vi "Dashboard Main.vi"() -> ()   [LabVIEW 2017]
uses:
  <vilib>/Utility/miscctls.llb/LVRowAndColumnTypeDef.ctl
  <vilib>/event_ctls.llb/eventvkey.ctl
  <vilib>/Rock Robotics/Network Tables/NT Read Numeric Array.vi
  <vilib>/Rock Robotics/WPI/Dashboard/WPI_DashboardLogging Global.vi
  <vilib>/Rock Robotics/Network Tables/NT Read Boolean.vi
panel:
  in  "Camera Settings Right":T1={"Frame Rate"=30, "Compression"=30, "Size"=1, "DB Camera Config"=FALSE} {"Frame Rate" scale=1.0..30.0; "Compression" scale=100.0..-1.0; "Size" items=["640x480", "320x240", "160x120"]}
  in  "Camera Name Right":string(combo)="No Camera Selection"
  out "Camera Info":cluster{"Mbps LED":bool, "Mbps":dbl, "fps":dbl} {"fps" format="%#.1g"; "Mbps" format="%#.1g"}
  in  "Camera Settings":T1={"Frame Rate"=30, "Compression"=30, "Size"=1, "DB Camera Config"=FALSE} {"Frame Rate" scale=1.0..30.0; "Compression" scale=100.0..-1.0; "Size" items=["640x480", "320x240", "160x120"]}
  in  "TCP":refnum<k5>
  in  "Rec Mode":enum32{"Stop", "Record", "Playback"}(radio)
  out "Robot IP":string
  out "Image Message":string="Timeout in Camera Communications"
  in  "Dashboard Tab":T2(tab)
  in  "Select Auto":string(combo)="Select Autonomous ..."
  out "NT Connection":bool
  out "MotorChart R":cluster{"Numeric":dbl, "Numeric":dbl}(graph)
  out "MotorChart L":cluster{"Numeric":dbl, "Numeric":dbl}(graph)
  out "MotorSliders R":cluster{"MotorSlide1":dbl, "MotorSlide2":dbl} {"MotorSlide2" scale=-1.0..1.0 scale format="%#_2e"; "MotorSlide1" scale=-1.0..1.0 scale format="%#_2e"}
  out "MotorSliders L":cluster{"MotorSlide1":dbl, "MotorSlide2":dbl} {"MotorSlide2" scale=-1.0..1.0 scale format="%#_2e"; "MotorSlide1" scale=-1.0..1.0 scale format="%#_2e"}
  out "Gyro":dbl(knob) scale=0.0..360.0
  out "JS1 Z":dbl(slide) scale=-1.0..1.0 scale format="%#_2e"
  out "JS1 Graph":cluster{"X":dbl, "Y":dbl}[](graph)
  out "JS1 Buttons":T3
  out "JS2 Z":dbl(slide) scale=-1.0..1.0 scale format="%#_2e"
  out "JS2 Graph":cluster{"X":dbl, "Y":dbl}[](graph)
  out "JS2 Buttons":T3
  out "Mode":T4(ring)=enum."Auto Disabled"
  out "Camera Image Right":T5(plugin-control)
  in  "DB/String 9":string
  in  "DB/String 8":string
  in  "DB/String 7":string
  in  "DB/String 6":string
  in  "DB/String 5":string
  in  "DB/String 4":string
  in  "DB/String 3":string
  in  "DB/String 2":string
  in  "DB/String 1":string
  in  "DB/String 0":string
  in  "DB/Slider 0":dbl(slide) scale=0.0..5.0
  in  "DB/Slider 1":dbl(slide) scale=0.0..5.0
  in  "DB/Slider 2":dbl(slide) scale=0.0..5.0
  in  "DB/Slider 3":dbl(slide) scale=0.0..5.0
  out "DB/LED 3":bool
  out "DB/LED 2":bool
  out "DB/LED 1":bool
  out "DB/LED 0":bool
  in  "DB/Button 3":bool
  in  "DB/Button 2":bool
  in  "DB/Button 1":bool
  in  "DB/Button 0":bool caption="New Name"
  out "Arm Error":string
  out "Has Cube":bool
  in  "Desired Elbow":dbl
  out "Error":string
  out "Shoulder":dbl
  out "Forearm":dbl
  in  "Desired Shoulder":dbl format="%#_13g"
  in  "Solenoid 1/Shoulder":bool
  in  "Solenoid 2/Forearm":bool
  in  "Test Slider":dbl(slide) scale=0.0..100.0 scale format="%#_3g"
  in  "On/Off":bool caption="Solenoid"
  in  "Test Name":u16(ring) items=["Select the test to run..."]
  in  "Test Tree":string(tree)
  in  "Motor":cluster{"Value":dbl, "Enable":bool} {"Value" scale=-1.0..1.0 scale format="%#_3g"}
  out "Progress":T6 {"Test Progress" scale=0.0..100.0}
  in  "Rev/Fwd":cluster{"Forward":bool, "Reverse":bool}
  in  "Test Ring":u16(ring) items=["Monochrome", "Color"]
  out "Cmd Status":string
  in  "Execute Command":bool
  in  "Command Params":string[][](table)
  in  "Command Selection":i32(listbox)
  in  "CheckList":i32(listbox)
  out "Tree":string(tree)
  out "Camera Image":T5(plugin-control)
  out "Background":bool
  in  "Camera Name":string(combo)="No Camera Selection"
  # "HW"
  # "HW"
  # "Joysticks"
  # "Drive Motors"
  # "Front"
  # "Right"
  # "Left"
  # "Back"
  # "This tab is a great place for autonomous settings and robot-specific values.\nPlace controls and indicators inside this tab and match name to\nDashboard Variables on robot. You can also delete this comment."
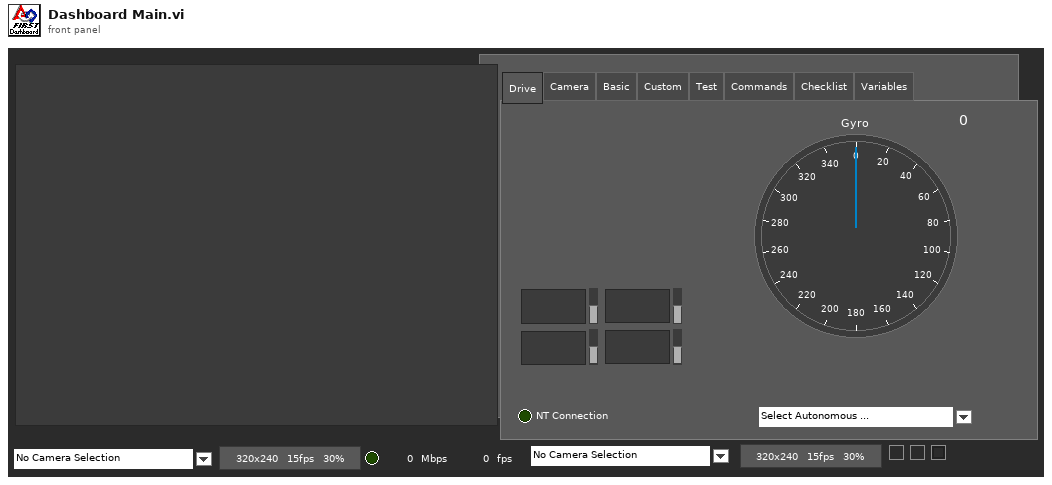
[diagram p1: front panel]
types:
  T1 = cluster{"Frame Rate":i32, "Compression":i32, "Size":u16, "DB Camera Config":bool}
  T2 = enum32{"Drive", "Camera", "Basic", "Custom", "Test", "Commands", "Checklist", "Variables"}
  T3 = cluster{bool, bool, bool, bool, bool, bool, bool, bool, bool, bool, bool, bool}
  T4 = enum8{"Tele-Op Disabled", "Tele-Op Enabled", "Auto Disabled", "Auto Enabled", "Test Disabled", "Test Enabled", "Disconnected", "No Code", "E-Stop"}
  T5 = typedef "IMAQ Image.ctl" = refnum<image>
  T6 = cluster{"Test Progress":u8, "Test Progress Text":string}
  T7 = cluster{"Save Path":path, "Interval (s)":dbl, "Keep":i32}
  T8 = typedef "Image Type" = u32
  T9 = cluster{"IDs":cluster{"RPC field ID":u16, "Unique ID":u16}, "String":string}
  T10 = cluster{"Error Strings":string, "Disable Counts":cluster{u16, u16}, "Rail Faults":cluster{u16, u16, u16}, "Robot IP":string, "DB Mode":u8, "Event Info":cluster{"Name":string, "Type":u8, "Number":u16, "Replay":u8}}
  T11 = cluster{"Storage":cluster{"Disk Free":u64, "RAM Block":u32, "RAM free":u32}, "CPU Utilization":cluster{"CPU % ISR":sgl, "CPU % Time Crit":sgl, "CPU % Timed Str":sgl, "CPU % High":sgl, "CPU % Above":sgl, "CPU % Normal":sgl, "CPU % Low":sgl}, "CAN":cluster{"% Bus Utilization":sgl, "Bus Off Cnt":u32, "TX_FIFO Full Cnt":u32, "Receive Error Cnt":u8, "Transmit Error Cnt":u8}, "HID":cluster{"HID Outputs":u32, "Rumble Low":u16, "Rumble High":u16}[]}
  T12 = cluster{"Status bits":cluster{"Test Mode":bool, "Autonomous":bool, "Enabled":bool, "Code Start":bool, "Brownout":bool, "Reserved 2":bool, "Reserved 3":bool, "E-Stop":bool}, "Code Trace":cluster{"Disabled":bool, "TeleOp":bool, "Auto":bool, "Test":bool}, "Controller Type":enum16{"unknown", "cRIO", "roboRio"}, "Code?":enum16{"unknown", "noCode", "code"}, "Battery V":dbl}
  T13 = cluster{"Control Bits":cluster{"TestMode":bool, "Autonomous":bool, "Enabled":bool, "FMS Present":bool, bool, bool, bool, "E-Stop":bool}, "Team Station ":u8, "Countdown":sgl, "Joystick Values":cluster{"Axes":dbl[], "Buttons":bool[], "POVs":i16[]}[]}
  T14 = cluster{"Axes":dbl[], "Buttons":bool[], "POVs":i16[]}[]
  T15 = cluster{"Axes":dbl[], "Buttons":bool[], "POVs":i16[]}
  T16 = cluster{"Buttons[0]":bool, "Buttons[1]":bool, "Buttons[2]":bool, "Buttons[3]":bool, "Buttons[4]":bool, "Buttons[5]":bool, "Buttons[6]":bool, "Buttons[7]":bool, "Buttons[8]":bool, "Buttons[9]":bool, "Buttons[10]":bool, "Buttons[11]":bool}
  T17 = cluster{"Camera Image":refnum<vi>, "Dashboard Tab":refnum<vi>, "Background":refnum<vi>, "Rec Mode":refnum<vi>, "Test Slider":refnum<vi>, "On/Off ":refnum<vi>, "Test Ring":refnum<vi>, "Rev/Fwd":refnum<vi>, "Test Name":refnum<vi>, "Motor":refnum<vi>, "Progress":refnum<vi>, "CheckList":refnum<vi>, "Tree":refnum<vi>, "Test Tree":refnum<vi>, "Command Params":refnum<vi>, "Command Selection":refnum<vi>, "Execute Command":refnum<vi>, "Cmd Status":refnum<vi>, "Camera Settings":refnum<vi>, "Camera Name":refnum<vi>, "Camera Info":refnum<vi>, "Camera Settings Right":refnum<vi>, "Camera Name Right":refnum<vi>, "Camera Image Right":refnum<vi>}
  T18 = cluster{"Camera Name Right":string, string, "Saved DB Images Info":cluster{"Save Path":path, "Interval (s)":dbl, "Keep":i32}}
  T19 = cluster{"Camera Name":string, string, "Saved DB Images Info":cluster{"Save Path":path, "Interval (s)":dbl, "Keep":i32}}
  T20 = cluster{"Operation":enum16{"Update", "Clear"}, "Color Box":u32}[]
  T21 = typedef "eventvkey.ctl" = enum16{"ASCII", "Enter", "Return", "Shift", "Ctrl", "Alt", "Cmd", "Opt", "Caps", "NumLock", "Clear", "Break", "Up", "Down", "Left", "Right", "Insert", "Delete", "Home", "End", "PageUp", "PageDown", "Escape", "Help", "Pause", "ScrollLock", "F1", "F2", "F3", "F4", "F5", "F6", "F7", "F8", "F9", "F10", "F11", "F12", "F13", "F14", "F15", "F16", "F17", "F18", "F19", "F20", "F21", "F22", "F23", "F24", "Play", "VolumeUp", "VolumeDown", "Mute", "Two Byte Char"}
  T22 = cluster{"Image Size":bool, "Image Type":bool, "Pixel Value":bool, "ROI Information":bool, "Zoom Factor":bool}
  T23 = cluster{"Operation":enum16{"Update", "Clear"}, "Color Box":u32}
  T24 = typedef "LVRowAndColumnTypeDef.ctl" = cluster{"Row":i32, "Column":i32}
  T25 = cluster{"Shift":bool, "Ctrl":bool, "Alt":bool, "Cmd":bool, "Opt":bool}
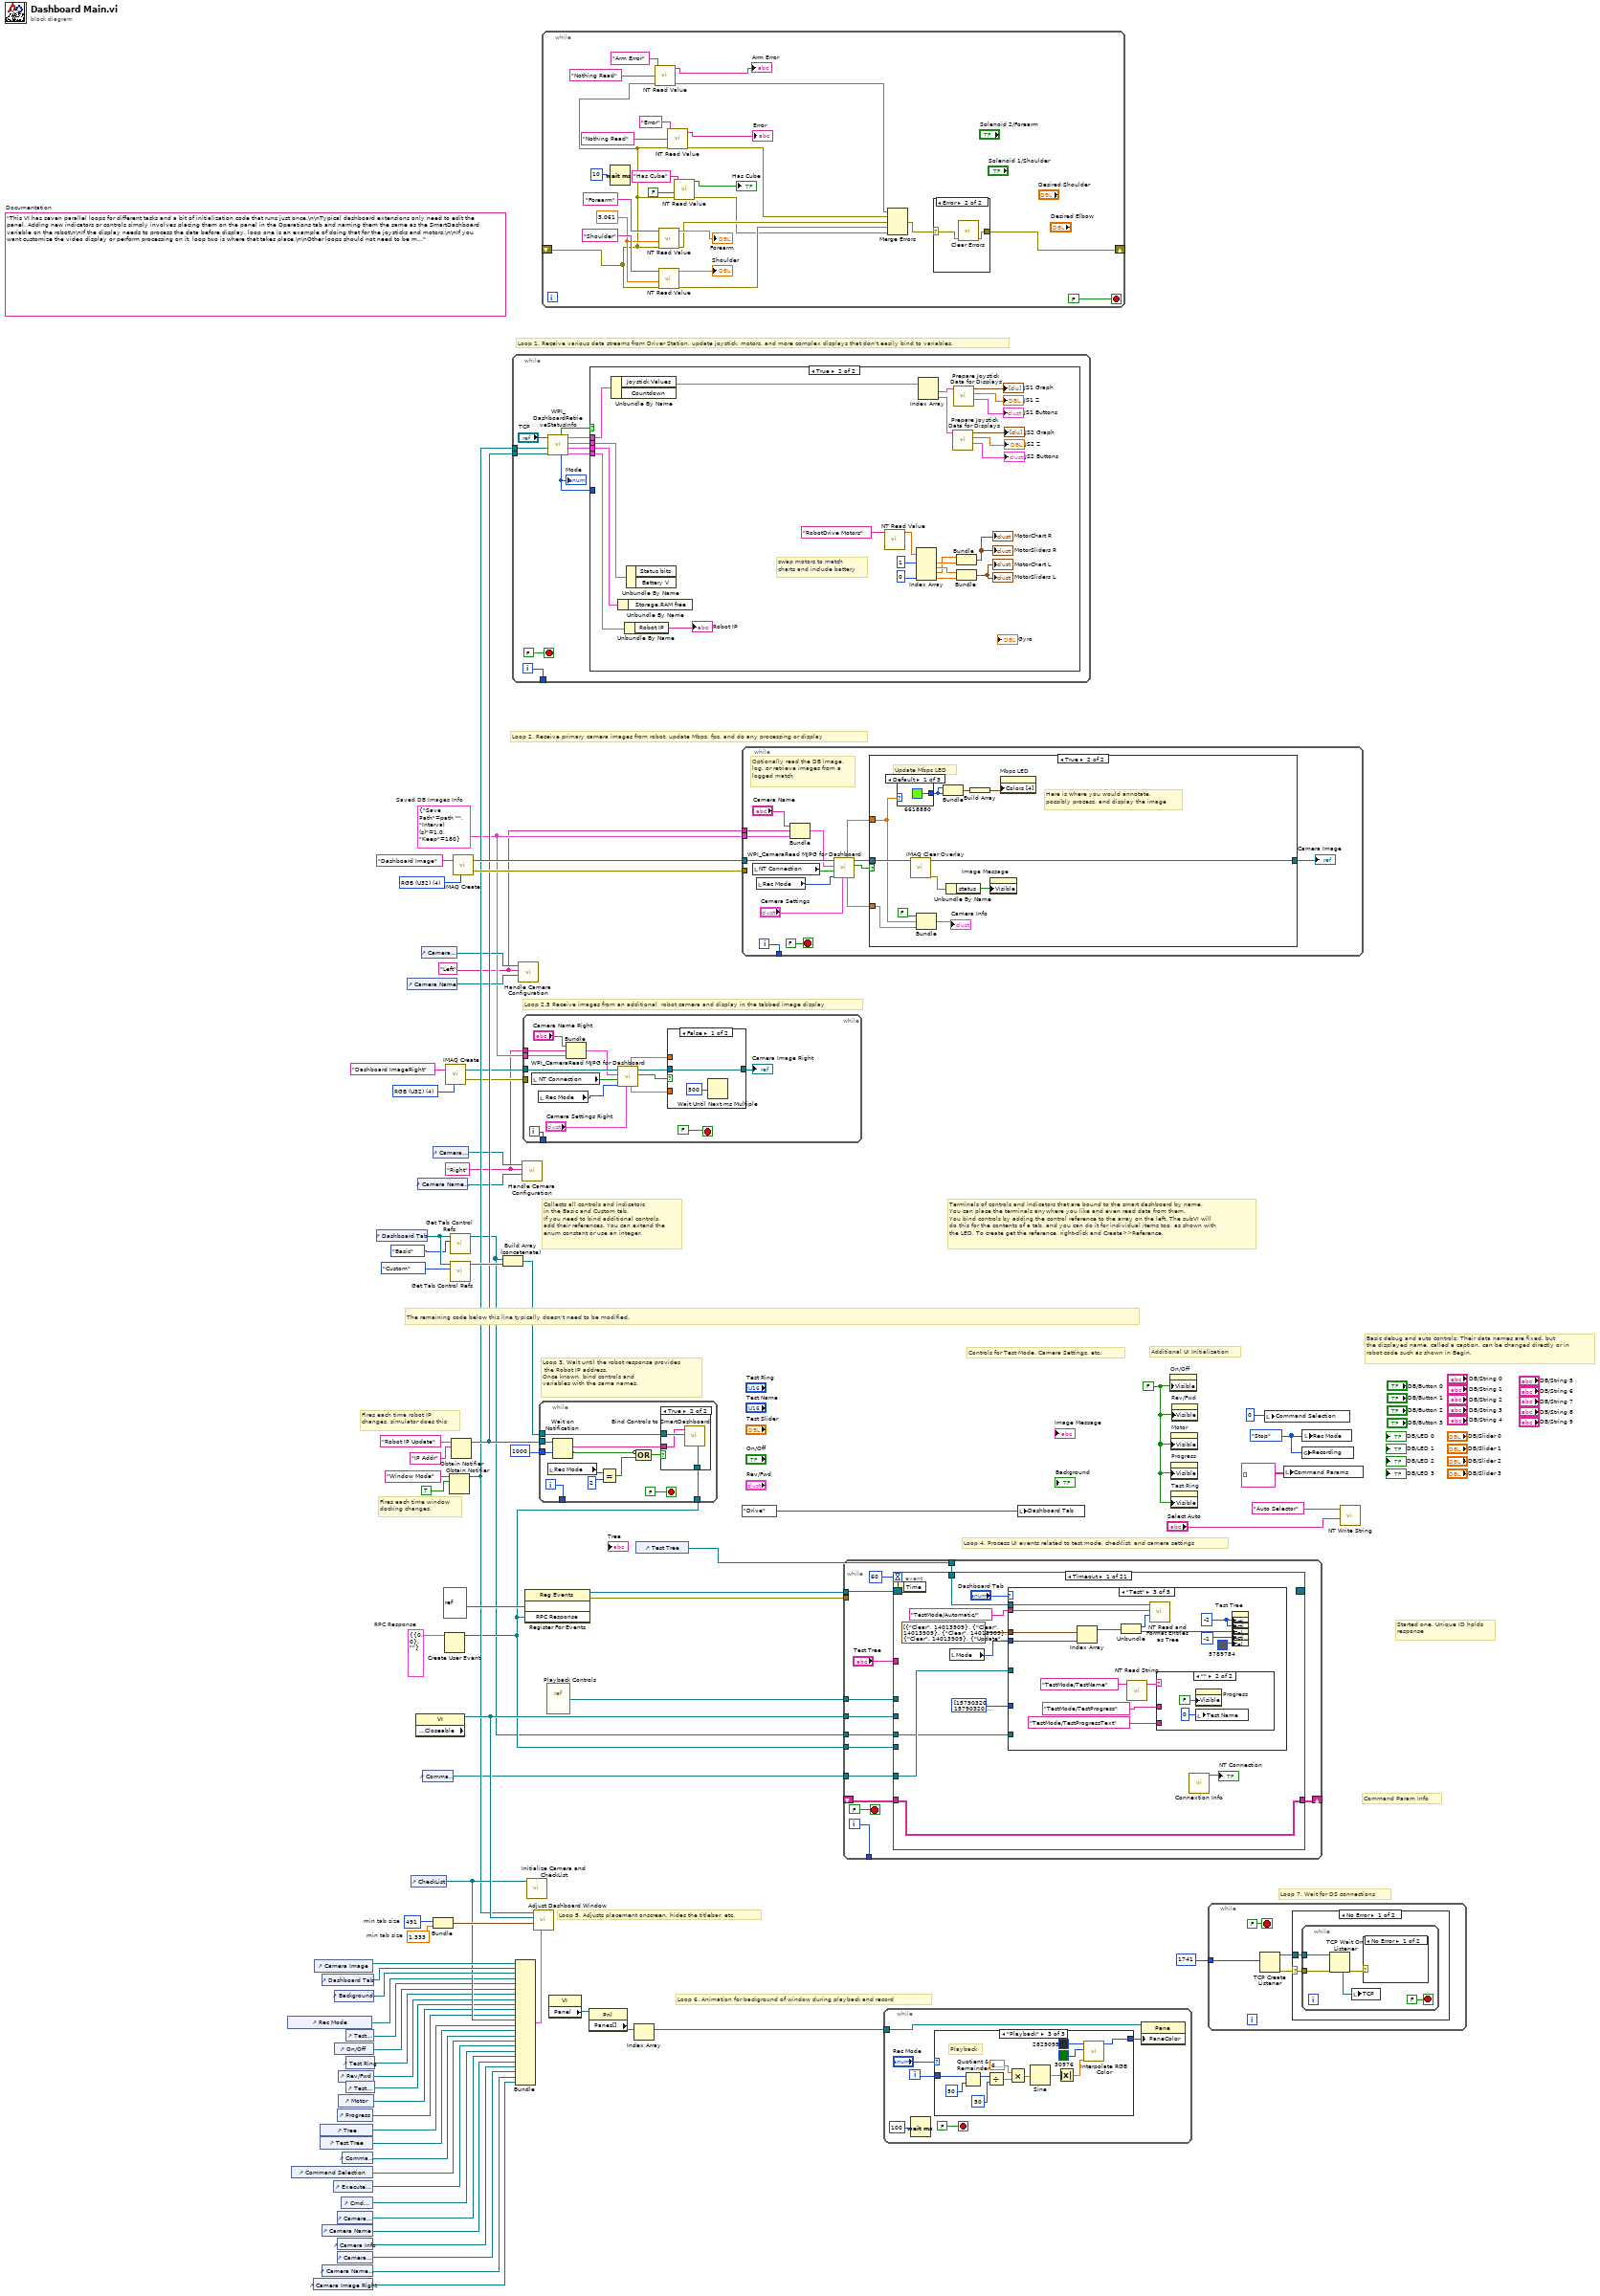
[diagram p0: block diagram]
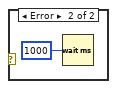
[diagram p4: hidden frame]
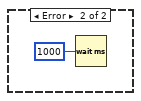
[diagram p5: hidden frame]
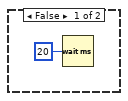
[diagram p6: hidden frame]
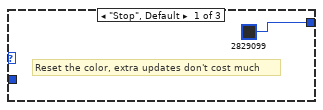
[diagram p7: hidden frame]
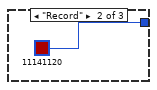
[diagram p8: hidden frame]
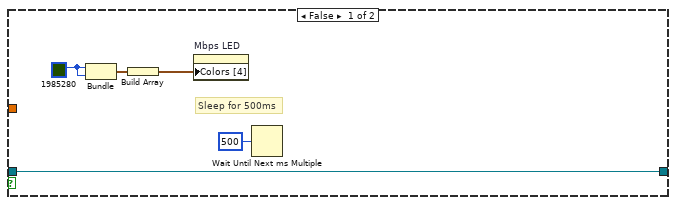
[diagram p10: hidden frame]
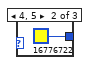
[diagram p11: hidden frame]
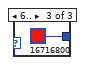
[diagram p12: hidden frame]
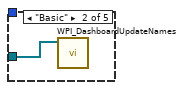
[diagram p14: hidden frame]
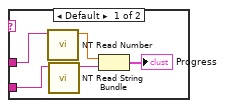
[diagram p15: hidden frame]
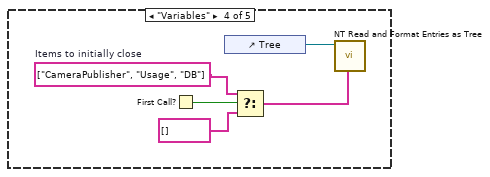
[diagram p16: hidden frame]
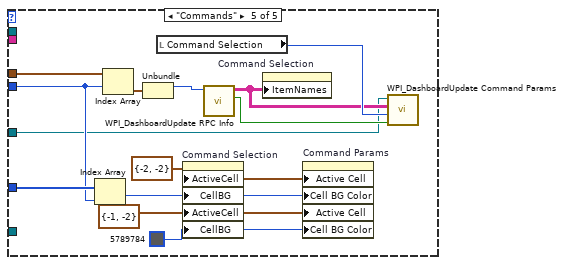
[diagram p17: hidden frame]
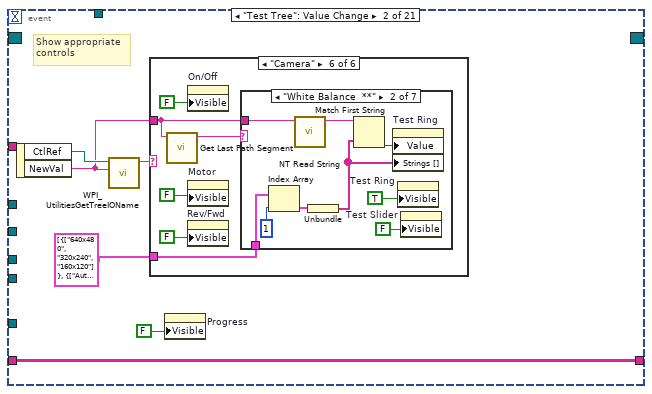
[diagram p18: hidden frame]
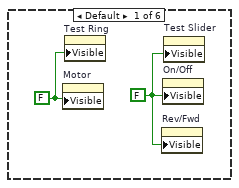
[diagram p19: hidden frame]
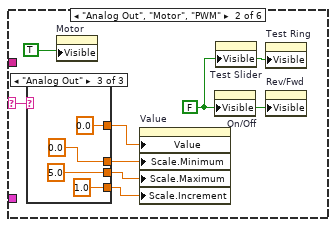
[diagram p20: hidden frame]
diagram:
  w3 = T7 {"Save Path"=path "", "Interval (s)"=1.0, "Keep"=180}  # Saved DB Images Info
  w2 = "Right"
  w1 = "Left"
  w13 = T8 4 items=["Grayscale (U8)", "Grayscale (I16)", "Grayscale (SGL)", "Complex (CSG)", "RGB (U32)", "HSL (U32)", "RGB (U64)"] ("Image Type")
  w29 = T9 {"IDs"={"RPC field ID"=0, "Unique ID"=0}, "String"=""}  # RPC Response
  w52 = 491  # min tab size
  w51 = 1.333  # min tab size
  w59 = enum32{"Stop", "Record", "Playback"}."Stop" ("Rec Mode")
  w36 = FALSE ("Visible")
  (unwired) "This VI has seven parallel loops for different tasks and a bit of initialization code that runs just once.\n\nTypical dashboard extensions only need to edit the panel. Adding new indicators or controls simply involves placing them on the panel in the Operations tab and naming them the same as the SmartDashboard variable on the robot\n\nIf the display needs to process the data before display, loop one is an example of doing that for the joysticks and motors.\n\nIf you want customize the video display or perform processing on it, loop two is where that takes place.\n\nOther loops should not need to be modified. They are pretty standard, and document the task they perform."  # Documentation
  w76 = T8 4 items=["Grayscale (U8)", "Grayscale (I16)", "Grayscale (SGL)", "Complex (CSG)", "RGB (U32)", "HSL (U32)", "RGB (U64)"] ("Image Type")
  # "Loop 2.5 Receive images from an additional  robot camera and display in the tabbed image display"
  # "Command Param Info"
  # "Started one, Unique ID holds\nresponse"
  # "Loop 7. Wait for DS connections"
  # "Basic debug and auto controls: Their data names are fixed, but\nthe displayed name, called a caption, can be changed directly or in\nrobot code such as shown in Begin."
  # "Controls for Test Mode, Camera Settings, etc."
  # "Additional UI Initialization"
  # "Loop 6. Animation for background of window during playback and record"
  # "Fires each time robot IP\nchanges, simulator does this"
  # "Fires each time window\ndocking changes."
  # "Collects all controls and indicators\nin the Basic and Custom tab.\nIf you need to bind additional controls,\nadd their references. You can extend the\nenum constant or use an integer."
  # "The remaining code below this line typically doesn't need to be modified."
  # "Loop 4. Process UI events related to test mode, checklist, and camera settings"
  # "Terminals of controls and indicators that are bound to the smart dashboard by name.\nYou can place the terminals anywhere you like and even read data from them.\nYou bind controls by adding the control reference to the array on the left. The subVI will\ndo this for the contents of a tab, and you can do it for individual items too, as shown with\nthe LED. To create get the reference, right-click and Create>>Reference."
  # "Loop 3. Wait until the robot response provides\n the Robot IP address.\nOnce known, bind controls and\nvariables with the same names."
  # "Loop 5. Adjusts placement onscreen, hides the titlebar, etc."
  # "Loop 1. Receive various data streams from Driver Station, update joystick, motors, and more complex displays that don't easily bind to variables."
  # "Loop 2. Receive primary camera images from robot, update Mbps, fps, and do any processing or display"
  n1 = control-ref of="Rec Mode"() -> (w42:refnum<vi>)
  n2 = control-ref of="Command Selection"() -> (w28:refnum<vi>)
  n3 = control-ref of="Camera Image Right"() -> (w6:refnum<vi>)
  n4 = control-ref of="Camera Image"() -> (w54:refnum<vi>)
  n5 = control-ref of="Tree"() -> (w46:refnum<vi>)
  n6 = control-ref of="Test Tree"() -> (w45:refnum<vi>)
  n7 = control-ref of="Dashboard Tab"() -> (w53:refnum<vi>)
  n8 = control-ref of="Camera Name"() -> (w19:refnum<vi>)
  n9 = control-ref of="Camera Name Right"() -> (w7:refnum<vi>)
  n10 = control-ref of="Execute Command"() -> (w30:refnum<vi>)
  n11 = control-ref of="Background"() -> (w49:refnum<vi>)
  n12 = control-ref of="On/Off"() -> (w40:refnum<vi>)
  n13 = control-ref of="Progress"() -> (w37:refnum<vi>)
  n14 = control-ref of="Camera Settings"() -> (w20:refnum<vi>)
  n15 = control-ref of="Camera Info"() -> (w18:refnum<vi>)
  n16 = control-ref of="Camera Settings Right"() -> (w8:refnum<vi>)
  n17 = control-ref of="Rev/Fwd"() -> (w38:refnum<vi>)
  n18 = control-ref of="Motor"() -> (w43:refnum<vi>)
  n19 = control-ref of="Cmd Status"() -> (w24:refnum<vi>)
  n20 = control-ref of="Command Params"() -> (w31:refnum<vi>)
  n21 = control-ref of="Test Slider"() -> (w41:refnum<vi>)
  n22 = control-ref of="Test Ring"() -> (w39:refnum<vi>)
  n23 = control-ref of="Test Name"() -> (w44:refnum<vi>)
  n24 = control-ref of="Dashboard Tab"() -> (w57:refnum<vi>)
  n25 = control-ref of="Camera Name"() -> (w21:refnum<vi>)
  n26 = control-ref of="CheckList"() -> (w47:refnum<vi>)
  n27 = property class="VI" props=["Front Panel.Closeable"]() -> (reference out=w58:refnum<vi>)  [unwired: 2 in, 2 out]
  n28 = control-ref of="Camera Name Right"() -> (w9:refnum<vi>)
  n29 = control-ref of="Camera Settings"() -> (w22:refnum<vi>)
  n30 = control-ref of="Command Params"() -> (w23:refnum<vi>)
  n31 = control-ref of="Camera Settings Right"() -> (w10:refnum<vi>)
  n32 = Bundle("min tab size"=w52, "min tab size"=w51) -> (w50:cluster{"min tab size":i32, "min tab size":dbl})  [unwired: 1 in]
  n33 = Create User Event(user event datatype=w29) -> (user event=w25:refnum<user-event>)  [unwired: 1 in, 1 out]
  n34 = call "IMAQ Create"("Image Name"="Dashboard ImageRight", "Image Type"=w13) -> ("New Image"=w12:T5, "error out"=w11:errorcluster)  [unwired: 2 in, 1 out]
  n35 = Obtain Notifier(name (unnamed)="Window Mode", notification data type=TRUE) -> (notifier out=w34:refnum<notifier>)  [unwired: 2 in, 2 out]
  n36 = call <vilib>:"Get Tab Control Refs.vi"("Page Index"=T2."Basic" ("Dashboard Tab"), "TabControl in"=w57) -> ("ControlsOnPage"=w17:refnum<vi>[])  [unwired: 9 in]
  n37 = call <vilib>:"Get Tab Control Refs.vi"("Page Index"=T2."Custom" ("Dashboard Tab"), "TabControl in"=w57) -> ("ControlsOnPage"=w56:refnum<vi>[])  [unwired: 9 in]
  n38 = Obtain Notifier(name (unnamed)="Robot IP Update", notification data type="IP Addr" ("name (unnamed)")) -> (notifier out=w35:refnum<notifier>)  [unwired: 2 in, 2 out]
  n39 = call "IMAQ Create"("Image Name"="Dashboard Image", "Image Type"=w76) -> ("New Image"=w74:T5, "error out"=w73:errorcluster)  [unwired: 2 in, 1 out]
  n40 = Build Array (concatenate)(w17, w56) -> (w55:refnum<vi>[])
  n41 = while {
    tunnel: [w86] -> _
    tunnel: w35 -> [w80]
    tunnel: w34 -> [w77]
    i -> [w86]
    stop <- FALSE stop-if-true
    n42 = call <vilib>:"WPI_DashboardRetrieveStatusInfo.vi"("Binding Refnum"=w80, "Window Mode Notifier"=w77, "TCP Cnx"="TCP") -> ("Power and Errors"=w81:T10, "Robot Metrics"=w84:T11, "Status Info"=w85:T12, "Control Info"=w82:T13, "Robot Mode"=w79:T4, "Process?"=w83:bool)  [unwired: 3 in]
    "Mode" <- w79
    n43 = case shown="True" w83 {
      tunnel: w85 -> [_ w112]
      tunnel: w84 -> [_ w111]
      tunnel: w82 -> [_ w110]
      tunnel: w81 -> [_ w109]
      tunnel: w79 -> [_ _]
      frame False {
        n44 = Wait (ms)(milliseconds to wait=u32 20) -> ()  [unwired: 1 out]
      }
      frame True {
        # "swap motors to match\ncharts and include battery"
        n45 = Unbundle By Name(w110) -> ("Joystick Values"=w100:T14)  [unwired: 1 out]
        n46 = Unbundle By Name(w111) -> ()  [unwired: 1 out]
        n47 = Unbundle By Name(w109) -> ("Robot IP"=→"Robot IP":string)
        n48 = Unbundle By Name(w112) -> ()  [unwired: 2 out]
        n49 = call-poly <vilib>:"NT Read Value.vi"("Name"="RobotDrive Motors") -> ("Numeric Array"=w90:dbl[])  [unwired: 9 in, 1 out]
        n50 = Index Array(array=w90, index #1=1, index #4=0) -> (element #1=w104:dbl, element #2=w105:dbl, element #3=w103:dbl, element #4=w108:dbl)  [unwired: 2 in]
        n51 = Index Array(array=w100) -> (element #1=w99:T15, element #2=w95:T15)  [unwired: 2 in]
        n52 = call "Prepare Joystick Data for Displays.vi"("Joystick Values"=w95) -> ("Buttons"=→"JS2 Buttons":T16, "Z Axis"=→"JS2 Z":dbl, "Cartesian Data"=→"JS2 Graph":cluster{"X axis":dbl, "X axis":dbl}[])  [unwired: 8 in]
        n53 = call "Prepare Joystick Data for Displays.vi"("Joystick Values"=w99) -> ("Buttons"=→"JS1 Buttons":T16, "Z Axis"=→"JS1 Z":dbl, "Cartesian Data"=→"JS1 Graph":cluster{"X axis":dbl, "X axis":dbl}[])  [unwired: 8 in]
        n54 = Bundle("Numeric"=w103, "Numeric"=w104) -> (→"MotorChart R" →"MotorSliders R":cluster{"Numeric":dbl, "Numeric":dbl})  [unwired: 1 in]
        n55 = Bundle("Numeric"=w105, "Numeric"=w108) -> (→"MotorChart L" →"MotorSliders L":cluster{"Numeric":dbl, "Numeric":dbl})  [unwired: 1 in]
      }
    }
  }
  n56 = Bundle("Camera Image"=w54, "Dashboard Tab"=w53, "Background"=w49, "Rec Mode"=w42, "Test Slider"=w41, "On/Off"=w40, "Test Ring"=w39, "Rev/Fwd"=w38, "Test Name"=w44, "Motor"=w43, "Progress"=w37, "CheckList"=w47, "Tree"=w46, "Test Tree"=w45, "Command Params"=w31, "Command Selection"=w28, "Execute Command"=w30, "Cmd Status"=w24, "Camera Settings"=w20, "Camera Name"=w19, "Camera Info"=w18, "Camera Settings Right"=w8, "Camera Name Right"=w7, "Camera Image Right"=w6) -> (w48:T17)  [unwired: 1 in]
  n57 = call "Handle Camera Configuration.vi"("CameraNameRef"=w21, "Display Name"=w1, "ClusterRef"=w22) -> ()  [unwired: 9 in]
  n58 = call "Handle Camera Configuration.vi"("CameraNameRef"=w9, "Display Name"=w2, "ClusterRef"=w10) -> ()  [unwired: 9 in]
  n59 = while {
    tunnel: w12 -> [w127]
    tunnel: w11 -> [_]
    tunnel: [w122] -> _
    tunnel: w3 -> [w116]
    tunnel: w2 -> [w113]
    i -> [w122]
    stop <- FALSE stop-if-true
    n60 = local read "NT Connection"() -> (w117:bool)
    n61 = local read "Rec Mode"() -> (w126:enum32{"Stop", "Record", "Playback"})
    n62 = Bundle("Camera Name Right"="Camera Name Right", w113, "Saved DB Images Info"=w116) -> (w115:T18)  [unwired: 1 in]
    n63 = call <vilib>:"WPI_CameraRead MJPG for Dashboard.vi"("Camera Settings"="Camera Settings Right", "Rec Mode"=w126, "NT Connection"=w117, "Capture Info"=w115, "Refnum in"=w127) -> ("Active"=w121:bool, "Refnum out"=w124:T5, "FPS"=w119:dbl, "Bandwidth (Mbps)"=w120:dbl)  [unwired: 3 in]
    n64 = case shown="False" w121 {
      tunnel: w124 -> [w128 w130]
      tunnel: w120 -> [_ _]
      tunnel: w119 -> [_ _]
      tunnel: [w128 w130] -> w118
      frame False {
        n65 = Wait Until Next ms Multiple(millisecond multiple=u32 500) -> ()  [unwired: 1 out]
      }
      frame True {
      }
    }
    "Camera Image Right" <- w118
  }
  n66 = register-events(refnum<vi> refnum, w25) -> (reference out=w63:refnum<event-registration>, error out=w62:errorcluster)  [unwired: 2 in]
  n67 = call "Initialize Camera and CheckList.vi"("ListBox in"=w47) -> ()  [unwired: 11 in]
  n68 = call "Adjust Dashboard Window.vi"("Sizing Refnums"=w48, "Size Constraints"=w50, "VI"=w58, "WIn Mode"=w34) -> ()  [unwired: 8 in]
  n69 = while {
    tunnel: w55 -> [w142]
    tunnel: w35 -> [w140]
    tunnel: [w138] -> _
    tunnel: u32 1000 ("milliseconds to wait") -> [w137]
    tunnel: w25 -> [w131]
    i -> [w138]
    stop <- FALSE stop-if-true
    n70 = local read "Rec Mode"() -> (w133:enum32{"Stop", "Record", "Playback"})
    n71 = Wait on Notification(notifier=w140, timeout in ms (-1)=w137) -> (notification=w139:string, timed out?=w135:bool)  [unwired: 2 in, 2 out]
    n72 = Equal?(x=w133, y=u16 2 ("Rec Mode")) -> (x = y?=w134:bool)
    n73 = Compound Arithmetic op=OR(invert w135, w134) -> (w136:bool)
    n74 = case shown="True" w136 {
      tunnel: w142 -> [_ w145]
      tunnel: w139 -> [_ w144]
      tunnel: w131 -> [_ w143]
      frame False {
      }
      frame True {
        n75 = call <vilib>:"Bind Controls to SmartDashboard.vi"("RPC ref"=w143, "Bound Control Refs"=w145, "Server IP Address"=w144) -> ()  [unwired: 9 in]
      }
    }
  }
  n76 = while {
    shift-right: [w155] -> _
    shift-left: _ -> [w146]
    stop <- FALSE stop-if-true
    w165 = 3.061 ("Default Value")
    n77 = Wait (ms)(milliseconds to wait=u32 10) -> ()  [unwired: 1 out]
    n78 = call-poly <vilib>:"NT Read Value.vi"("error in"=w146, "Default Value"="Nothing Read", "Name"="Arm Error") -> ("error out"=w147:errorcluster, "String"=→"Arm Error":string)  [unwired: 7 in]
    n79 = call-poly <vilib>:"NT Read Value.vi"("error in"=w146, "Default Value"=w165, "Name"="Forearm") -> ("error out"=w164:errorcluster, "Numeric"=→"Forearm":dbl)  [unwired: 7 in]
    n80 = call-poly <vilib>:"NT Read Value.vi"("error in"=w146, "Default Value"=w165, "Name"="Shoulder") -> ("error out"=w163:errorcluster, "Numeric"=→"Shoulder":dbl)  [unwired: 7 in]
    n81 = call-poly <vilib>:"NT Read Value.vi"("error in"=w146, "Default Value"="Nothing Read", "Name"="Error") -> ("error out"=w158:errorcluster, "String"=→"Error":string)  [unwired: 7 in]
    n82 = call-poly <vilib>:"NT Read Value.vi"("error in"=w146, "Default Value"=FALSE, "Name"="Has Cube") -> ("error out"=w151:errorcluster, "Boolean"=→"Has Cube":bool)  [unwired: 7 in]
    n83 = Merge Errors(w147, w158, w164, w163, w151) -> (w156:errorcluster)
    n84 = case shown="Error" w156 {
      selector: w156 -> [w170 w172]
      tunnel: [w170 w171] -> w155
      frame No Error {
      }
      frame Error {
        n85 = call <vilib>:"Clear Errors.vi"("error in (no error)"=w172) -> ("error out"=w171:errorcluster)  [unwired: 5 in, 1 out]
      }
    }
  }
  n86 = vi-ref "Playback Controls.vi"() -> (w64:refnum<vi>)
  n87 = property class="VI"() -> ("Panel"=w66:refnum<vi>)  [unwired: 2 in, 2 out]
  n88 = property class="Pnl"(reference=w66) -> ("Panes[]"=w67:refnum<vi>[])  [unwired: 1 in, 2 out]
  n89 = Index Array(array=w67) -> (element=w65:refnum<vi>)  [unwired: 1 in]
  n90 = control-ref of="Test Tree"() -> (w68:refnum<vi>)
  n91 = while {
    tunnel: w74 -> [w185]
    tunnel: w73 -> [_]
    tunnel: [w186] -> _
    tunnel: w3 -> [w176]
    tunnel: w1 -> [w173]
    i -> [w186]
    stop <- FALSE stop-if-true
    # "Optionally read the DB image,\nlog, or retrieve images from a\nlogged match"
    n92 = local read "NT Connection"() -> (w177:bool)
    n93 = local read "Rec Mode"() -> (w181:enum32{"Stop", "Record", "Playback"})
    n94 = Bundle("Camera Name"="Camera Name", w173, "Saved DB Images Info"=w176) -> (w175:T19)  [unwired: 1 in]
    n95 = call <vilib>:"WPI_CameraRead MJPG for Dashboard.vi"("Camera Settings"="Camera Settings", "Rec Mode"=w181, "NT Connection"=w177, "Capture Info"=w175, "Refnum in"=w185) -> ("Active"=w183:bool, "Refnum out"=w184:T5, "FPS"=w182:dbl, "Bandwidth (Mbps)"=w180:dbl)  [unwired: 3 in]
    n96 = case shown="True" w183 {
      tunnel: w184 -> [w188 w199]
      tunnel: w180 -> [_ w196]
      tunnel: w182 -> [_ w197]
      tunnel: [w188 w193] -> w178
      frame False {
        w190 = u32 1985280 ("Color Box")
        # "Sleep for 500ms"
        n97 = Bundle("Color Box"=w190, "Color Box"=w190) -> (w191:cluster{"Color Box":u32, "Color Box":u32})  [unwired: 1 out]
        n98 = Build Array(w191) -> (w189:cluster{"Color Box":u32, "Color Box":u32}[])
        n99 = property on="Mbps LED" class="Bool (strict)"("Colors [4]"=w189) -> ()  [unwired: 2 in, 2 out]
        n100 = Wait Until Next ms Multiple(millisecond multiple=u32 500) -> ()  [unwired: 1 out]
      }
      frame True {
        # "Here is where you would annotate,\npossibly process, and display the image"
        # "Update Mbps LED"
        n101 = case shown="Default" w196 {
          tunnel: [u32 6618880 ("Color Box") u32 16776722 ("Color Box") u32 16716800 ("Color Box")] -> w200
          frame Default {
          }
          frame 4, 5 {
          }
          frame 6.. {
          }
        }
        n102 = call "IMAQ Clear Overlay"("Image"=w199) -> ("error out"=w202:errorcluster, "Image Out"=w193:T5)  [unwired: 2 in, 7 out]
        n103 = Bundle(FALSE, "Bandwidth (Mbps)"=w196, "FPS"=w197) -> (→"Camera Info":cluster{bool, "Bandwidth (Mbps)":dbl, "FPS":dbl})  [unwired: 1 in]
        n104 = Bundle("Color Box"=w200, "Color Box"=w200) -> (w201:cluster{"Color Box":u32, "Color Box":u32})  [unwired: 1 out]
        n105 = Unbundle By Name(w202) -> ("status"=w203:bool)
        n106 = Build Array(w201) -> (w198:cluster{"Color Box":u32, "Color Box":u32}[])
        n107 = property on="Image Message" class="Str"("Visible"=w203) -> ()  [unwired: 2 in, 2 out]
        n108 = property on="Mbps LED" class="Bool (strict)"("Colors [4]"=w198) -> ()  [unwired: 2 in, 2 out]
      }
    }
    "Camera Image" <- w178
  }
  n109 = while {
    tunnel: [w216] -> _
    tunnel: w68 -> [w215]
    tunnel: w64 -> [w214]
    tunnel: w63 -> [w213]
    tunnel: w62 -> [_]
    tunnel: w58 -> [w212]
    tunnel: w25 -> [w211]
    tunnel: w23 -> [w210]
    shift-right: [w209] -> _
    shift-left: _ -> [w208]
    tunnel: w17 -> [w207]
    i -> [w216]
    stop <- FALSE stop-if-true
    n110 = event shown="[0] Timeout" {
      selector: w213 -> [_ _ _ _ _ _ _ _ _ _ _ _ _ _ _ _ _ _ _ _ _]
      dyn-events: [_ _ _ _ _ _ _ _ _ _ _ _ _ _ _ _ w476 _ _ _ _] -> _
      timeout: u32 60 ("milliseconds to wait") -> [_ _ _ _ _ _ _ _ _ _ _ _ _ _ _ _ _ _ _ _ _]
      tunnel: w215 -> [w228 _ _ _ _ _ _ _ _ _ _ _ _ _ _ _ _ _ _ _ _]
      tunnel: "Test Tree" -> [_ _ _ _ _ _ _ _ _ _ _ w443 w451 w453 w457 w465 _ _ _ _ _]
      tunnel: w214 -> [_ _ _ _ _ _ _ _ _ _ _ _ _ _ _ _ w478 _ w496 _ _]
      tunnel: w212 -> [_ _ _ _ _ _ _ _ _ _ _ _ _ _ _ _ w474 _ _ _ _]
      tunnel: w211 -> [_ _ _ _ _ _ _ _ _ _ _ _ _ _ _ _ w472 _ _ _ _]
      tunnel: w210 -> [w223 _ _ _ _ _ w394 _ _ _ _ _ _ _ _ _ _ _ _ _ _]
      tunnel: [w222 w271 w373 w378 w387 w391 w392 w401 w411 w418 w430 w442 w449 w452 w456 w464 w471 w491 w493 w497 w510] -> w209
      tunnel: w208 -> [w222 w271 w373 w378 w387 w391 w392 _ _ w418 w430 w442 w449 w452 w456 w464 w471 w491 w493 w497 w510]
      tunnel: w207 -> [w220 _ _ _ _ _ _ _ _ _ _ _ _ _ _ _ _ _ _ _ _]
      event Timeout {
        n111 = event-data() -> ()  [unwired: 1 in, 1 out]
        n112 = local read "Mode"() -> (w225:T4)
        n113 = case shown="\"Test\"" "Dashboard Tab" {
          tunnel: w228 -> [_ _ w244 _ _]
          tunnel: "TestMode/Automatic/" ("Name Pattern") -> [_ _ w243 _ _]
          tunnel: T20 [{"Operation"=enum."Clear", "Color Box"=14013909}, {"Operation"=enum."Clear", "Color Box"=14013909}, {"Operation"=enum."Clear", "Color Box"=14013909}, {"Operation"=enum."Clear", "Color Box"=14013909}, {"Operation"=enum."Update", "Color Box"=14013909}, {"Operation"=enum."Update", "Color Box"=16777215}, {"Operation"=enum."Clear", "Color Box"=14013909}, {"Operation"=enum."Clear", "Color Box"=14013909}, {"Operation"=enum."Clear", "Color Box"=14013909}] -> [_ _ w236 _ w264]
          tunnel: w225 -> [_ _ w235 _ w263]
          tunnel: u32[] [15790320, 15790320, 15790320, 15790320, 16777215, 16777215, 15790320, 15790320, 15790320] -> [_ _ _ _ w269]
          tunnel: w223 -> [_ _ _ _ w257]
          tunnel: w220 -> [_ w230 _ _ _]
          frame "Custom", Default {
          }
          frame "Basic" {
            n114 = call <vilib>:"WPI_DashboardUpdateNames.vi"("Controls on Tab"=w230) -> ()  [unwired: 11 in]
          }
          frame "Test" {
            w242 = -2 ("Active Item:Row Number")
            n115 = Index Array(array=w236, index=w235) -> (element=w237:T23)
            n116 = Unbundle(w237) -> ("Operation"=w238:enum16{"Update", "Clear"}, "Color Box"=w239:u32)
            n117 = call <vilib>:"NT Read String.vi"("Name"="TestMode/TestName") -> ("String"=w233:string)  [unwired: 9 in, 1 out]
            n118 = call <vilib>:"NT Read and Format Entries as Tree.vi"("Operation"=w238, "Name Pattern"=w243, "Tree Refnum"=w244) -> ()  [unwired: 7 in, 2 out]
            n119 = case shown="\"\"" w233 {
              tunnel: "TestMode/TestProgress" ("Name") -> [w246 _]
              tunnel: "TestMode/TestProgressText" ("Name") -> [w245 _]
              frame Default {
                n120 = call <vilib>:"NT Read Number.vi"("Name"=w246) -> ("Numeric"=w247:dbl)  [unwired: 9 in, 1 out]
                n121 = call <vilib>:"NT Read String.vi"("Name"=w245) -> ("String"=w248:string)  [unwired: 9 in, 1 out]
                n122 = Bundle("Numeric"=w247, "String"=w248) -> (→"Progress":cluster{"Numeric":dbl, "String":string})  [unwired: 1 in]
              }
              frame "" {
                n123 = property on="Progress" class="Clust (strict)"("Visible"=FALSE) -> ()  [unwired: 2 in, 2 out]
                n124 = local write "Test Name"(u16 0) -> ()
              }
            }
            n125 = property on="Test Tree" class="Tree (strict)"("Active Item Row Number"=w242, "ActiveColNum"=w242, "CellBG"=w239, "Active Item Row Number"=-1 ("Active Item:Row Number"), "CellBG"=u32 5789784 ("Color Box")) -> ()  [unwired: 2 in, 2 out]
          }
          frame "Variables" {
            w254 = string[] ["CameraPublisher", "Usage", "DB"]  # Items to initially close
            n126 = First Call?() -> (First Call?: T/F=w255:bool)
            n127 = control-ref of="Tree"() -> (w256:refnum<vi>)
            n128 = Select(t=w254, s=w255, f=string[] []) -> (s? t:f=w252:string[])
            n129 = call <vilib>:"NT Read and Format Entries as Tree.vi"("Tags to  Close"=w252, "Tree Refnum"=w256) -> ()  [unwired: 8 in, 2 out]
          }
          frame "Commands" {
            w265 = u32 5789784 ("Color Box")
            w266 = T24 {"Row"=-1, "Column"=-2} ("Active Cell:Active Cell")
            w268 = T24 {"Row"=-2, "Column"=-2} ("Active Cell:Active Cell")
            n130 = Index Array(array=w269, index=w263) -> (element=w267:u32)
            n131 = Index Array(array=w264, index=w263) -> (element=w262:T23)
            n132 = Unbundle(w262) -> ("Operation"=w261:enum16{"Update", "Clear"})  [unwired: 1 out]
            n133 = local read "Command Selection"() -> (w260:i32)
            n134 = property on="Command Selection" class="MCListbox (strict)"("ActiveCell"=w268, "CellBG"=w267, "ActiveCell"=w266, "CellBG"=w265) -> ()  [unwired: 2 in, 2 out]
            n135 = call <vilib>:"WPI_DashboardUpdate RPC Info.vi"("Operation"=w261) -> ("update"=w259:bool, "commands"=w258:string[][])  [unwired: 9 in]
            n136 = property on="Command Selection" class="MCListbox (strict)"("ItemNames"=w258) -> ()  [unwired: 2 in, 2 out]
            n137 = property on="Command Params" class="Tbl (strict)"("Active Cell"=w268, "Cell BG Color"=w267, "Active Cell"=w266, "Cell BG Color"=w265) -> ()  [unwired: 2 in, 2 out]
            n138 = call <vilib>:"WPI_DashboardUpdate Command Params.vi"("Update"=w259, "NewVal"=w260, "Commands"=w258, "Param Tbl"=w257) -> ()  [unwired: 7 in, 1 out]
          }
        }
        n139 = call <vilib>:"Connextion Info.vi"() -> ("Connected"=→"NT Connection":bool)  [unwired: 10 in, 1 out]
      }
      event "Test Tree": Value Change {
        # "Show appropriate\ncontrols"
        n140 = event-data() -> ("CtlRef"=w274:refnum<vi>, "NewVal"=w272:string)  [unwired: 1 in]
        n141 = call <vilib>:"WPI_UtilitiesGetTreeIOName.vi"("NewVal"=w272, "TreeControl in"=w274) -> ("I/O Name"=w275:string)  [unwired: 9 in]
        n142 = case shown="\"Camera\"" w275 {
          selector: w275 -> [_ w282 _ w304 w313 _]
          tunnel: w272 -> [_ _ w301 w303 _ w320]
          tunnel: cluster{string[]}[] [{["640x480", "320x240", "160x120"]}, {["Auto", "Fixed indoor", "Fixed outdoor 1", "Fixed outdoor 2", "Fixed fluorescent 1", "Fixed fluorescent 2", "Hold current"]}, {["Auto", "Flicker-free 50 Hz", "Flicker-free 60 Hz", "Hold current"]}, {["None", "Prioritize frame rate", "Prioritize image quality"]}, {["Monochrome", "Color"]}] -> [_ _ _ _ _ w319]
          frame Default {
            w277 = FALSE ("Visible")
            w276 = FALSE ("Visible")
            n143 = property on="Motor" class="Clust (strict)"("Visible"=w276) -> ()  [unwired: 2 in, 2 out]
            n144 = property on="Test Ring" class="Ring (strict)"("Visible"=w276) -> ()  [unwired: 2 in, 2 out]
            n145 = property on="Rev/Fwd" class="Clust (strict)"("Visible"=w277) -> ()  [unwired: 2 in, 2 out]
            n146 = property on="On/Off" class="Bool (strict)"("Visible"=w277) -> ()  [unwired: 2 in, 2 out]
            n147 = property on="Test Slider" class="Slide (strict)"("Visible"=w277) -> ()  [unwired: 2 in, 2 out]
          }
          frame "Analog Out", "Motor", "PWM" {
            w283 = FALSE ("Visible")
            n148 = case shown="\"Analog Out\"" w282 {
              tunnel: [1.0 ("Value") -1.0 ("Value") 0.0 ("Value")] -> w281
              tunnel: [255.0 ("Value") 1.0 ("Value") 5.0 ("Value")] -> w280
              tunnel: [128.0 ("Value") 0.0 ("Value") 0.0 ("Value")] -> w279
              tunnel: [64.0 ("Value") 0.5 ("Value") 1.0 ("Value")] -> w278
              frame "PWM" {
              }
              frame "Motor", Default {
              }
              frame "Analog Out" {
              }
            }
            n149 = property on="Motor" class="Clust (strict)"("Visible"=TRUE) -> ()  [unwired: 2 in, 2 out]
            n150 = property on="Value" class="Slide (strict)"("Value"=w279, "Scale.Minimum"=w281, "Scale.Maximum"=w280, "Scale.Increment"=w278) -> ()  [unwired: 2 in, 2 out]
            n151 = property on="On/Off" class="Bool (strict)"("Visible"=w283) -> ()  [unwired: 2 in, 2 out]
            n152 = property on="Test Slider" class="Slide (strict)"("Visible"=w283) -> ()  [unwired: 2 in, 2 out]
            n153 = property on="Test Ring" class="Ring (strict)"("Visible"=w283) -> ()  [unwired: 2 in, 2 out]
            n154 = property on="Rev/Fwd" class="Clust (strict)"("Visible"=w283) -> ()  [unwired: 2 in, 2 out]
          }
          frame "Servo" {
            w299 = FALSE ("Visible")
            n155 = call <vilib>:"NT Read Number.vi"("Name"=w301) -> ("Numeric"=w300:dbl)  [unwired: 9 in, 1 out]
            n156 = property on="Test Slider" class="Slide (strict)"("Visible"=TRUE, "Scale.Maximum"=170.0 ("Scale.Range:Maximum")) -> ()  [unwired: 2 in, 2 out]
            n157 = local write "Test Slider"(w300) -> ()
            n158 = property on="Motor" class="Clust (strict)"("Visible"=w299) -> ()  [unwired: 2 in, 2 out]
            n159 = property on="Rev/Fwd" class="Clust (strict)"("Visible"=w299) -> ()  [unwired: 2 in, 2 out]
            n160 = property on="On/Off" class="Bool (strict)"("Visible"=w299) -> ()  [unwired: 2 in, 2 out]
            n161 = property on="Test Ring" class="Ring (strict)"("Visible"=w299) -> ()  [unwired: 2 in, 2 out]
          }
          frame "Relay", "Solenoid" {
            w302 = FALSE ("Visible")
            n162 = property on="Motor" class="Clust (strict)"("Visible"=w302) -> ()  [unwired: 2 in, 2 out]
            n163 = property on="Test Slider" class="Slide (strict)"("Visible"=w302) -> ()  [unwired: 2 in, 2 out]
            n164 = Search and Replace String(input string=w303, search string="/Value  **", replace string="/Direction") -> (result string=w309:string)  [unwired: 5 in, 3 out]
            n165 = property on="Test Ring" class="Ring (strict)"("Visible"=w302) -> ()  [unwired: 2 in, 2 out]
            n166 = call <vilib>:"NT Read String.vi"("Name"=w309) -> ("String"=w307:string)  [unwired: 9 in, 1 out]
            n167 = Equal?(x="Both directions", y=w307) -> (x = y?=w305:bool)
            n168 = Not(x=w305) -> (.not. x?=w306:bool)
            n169 = property on="Rev/Fwd" class="Clust (strict)"("Visible"=w305) -> ()  [unwired: 2 in, 2 out]
            n170 = property on="On/Off" class="Bool (strict)"("Visible"=w306, "Caption.Text"=w304) -> ()  [unwired: 2 in, 2 out]
          }
          frame "Compressor", "Digital Out" {
            w312 = FALSE ("Visible")
            # "Get direction and finish"
            n171 = property on="Motor" class="Clust (strict)"("Visible"=w312) -> ()  [unwired: 2 in, 2 out]
            n172 = property on="Test Slider" class="Slide (strict)"("Visible"=w312) -> ()  [unwired: 2 in, 2 out]
            n173 = property on="Test Ring" class="Ring (strict)"("Visible"=w312) -> ()  [unwired: 2 in, 2 out]
            n174 = property on="On/Off" class="Bool (strict)"("Visible"=TRUE, "Caption.Text"=w313) -> ()  [unwired: 2 in, 2 out]
            n175 = property on="Rev/Fwd" class="Clust (strict)"("Visible"=FALSE) -> ()  [unwired: 2 in, 2 out]
          }
          frame "Camera" {
            n176 = call <vilib>:"Get Last Path Segment.vi"("String in"=w320) -> ("String out"=w321:string)  [unwired: 10 in]
            n177 = property on="On/Off" class="Bool (strict)"("Visible"=FALSE) -> ()  [unwired: 2 in, 2 out]
            n178 = property on="Motor" class="Clust (strict)"("Visible"=FALSE) -> ()  [unwired: 2 in, 2 out]
            n179 = property on="Rev/Fwd" class="Clust (strict)"("Visible"=FALSE) -> ()  [unwired: 2 in, 2 out]
            n180 = case shown="\"White Balance  **\"" w321 {
              tunnel: w320 -> [w327 w336 w345 w354 w363 _ w369]
              tunnel: w319 -> [w325 w333 w342 w351 w360 _ _]
              frame "Size  **" {
                n181 = Index Array(array=w325) -> (element=w324:cluster{string[]})  [unwired: 1 in]
                n182 = call <vilib>:"NT Read String.vi"("Name"=w327) -> ("String"=w326:string)  [unwired: 9 in, 1 out]
                n183 = Unbundle(w324) -> (w322:string[])
                n184 = Match First String(2:w322, 3:w326) -> (0:w323:i32)  [unwired: 1 out]
                n185 = property on="Test Ring" class="Ring (strict)"("Value"=w323, "Strings []"=w322) -> ()  [unwired: 2 in, 2 out]
                n186 = property on="Test Ring" class="Ring (strict)"("Visible"=TRUE) -> ()  [unwired: 2 in, 2 out]
                n187 = property on="Test Slider" class="Slide (strict)"("Visible"=FALSE) -> ()  [unwired: 2 in, 2 out]
              }
              frame "White Balance  **" {
                n188 = Index Array(array=w333, index=1) -> (element=w334:cluster{string[]})
                n189 = call <vilib>:"NT Read String.vi"("Name"=w336) -> ("String"=w335:string)  [unwired: 9 in, 1 out]
                n190 = Unbundle(w334) -> (w331:string[])
                n191 = Match First String(2:w331, 3:w335) -> (0:w330:i32)  [unwired: 1 out]
                n192 = property on="Test Ring" class="Ring (strict)"("Value"=w330, "Strings []"=w331) -> ()  [unwired: 2 in, 2 out]
                n193 = property on="Test Ring" class="Ring (strict)"("Visible"=TRUE) -> ()  [unwired: 2 in, 2 out]
                n194 = property on="Test Slider" class="Slide (strict)"("Visible"=FALSE) -> ()  [unwired: 2 in, 2 out]
              }
              frame "Exposure  **" {
                n195 = Index Array(array=w342, index=2) -> (element=w343:cluster{string[]})
                n196 = call <vilib>:"NT Read String.vi"("Name"=w345) -> ("String"=w344:string)  [unwired: 9 in, 1 out]
                n197 = Unbundle(w343) -> (w339:string[])
                n198 = Match First String(2:w339, 3:w344) -> (0:w340:i32)  [unwired: 1 out]
                n199 = property on="Test Ring" class="Ring (strict)"("Value"=w340, "Strings []"=w339) -> ()  [unwired: 2 in, 2 out]
                n200 = property on="Test Ring" class="Ring (strict)"("Visible"=TRUE) -> ()  [unwired: 2 in, 2 out]
                n201 = property on="Test Slider" class="Slide (strict)"("Visible"=FALSE) -> ()  [unwired: 2 in, 2 out]
              }
              frame "Exposure Priority  **" {
                n202 = Index Array(array=w351, index=3) -> (element=w352:cluster{string[]})
                n203 = call <vilib>:"NT Read String.vi"("Name"=w354) -> ("String"=w353:string)  [unwired: 9 in, 1 out]
                n204 = Unbundle(w352) -> (w348:string[])
                n205 = Match First String(2:w348, 3:w353) -> (0:w349:i32)  [unwired: 1 out]
                n206 = property on="Test Ring" class="Ring (strict)"("Value"=w349, "Strings []"=w348) -> ()  [unwired: 2 in, 2 out]
                n207 = property on="Test Ring" class="Ring (strict)"("Visible"=TRUE) -> ()  [unwired: 2 in, 2 out]
                n208 = property on="Test Slider" class="Slide (strict)"("Visible"=FALSE) -> ()  [unwired: 2 in, 2 out]
              }
              frame "Color Enable  **" {
                n209 = Index Array(array=w360, index=4) -> (element=w361:cluster{string[]})
                n210 = call <vilib>:"NT Read String.vi"("Name"=w363) -> ("String"=w362:string)  [unwired: 9 in, 1 out]
                n211 = Unbundle(w361) -> (w357:string[])
                n212 = Match First String(2:w357, 3:w362) -> (0:w358:i32)  [unwired: 1 out]
                n213 = property on="Test Ring" class="Ring (strict)"("Value"=w358, "Strings []"=w357) -> ()  [unwired: 2 in, 2 out]
                n214 = property on="Test Ring" class="Ring (strict)"("Visible"=TRUE) -> ()  [unwired: 2 in, 2 out]
                n215 = property on="Test Slider" class="Slide (strict)"("Visible"=FALSE) -> ()  [unwired: 2 in, 2 out]
              }
              frame Default {
                n216 = property on="Test Ring" class="Ring (strict)"("Visible"=FALSE) -> ()  [unwired: 2 in, 2 out]
                n217 = property on="Test Slider" class="Slide (strict)"("Visible"=FALSE) -> ()  [unwired: 2 in, 2 out]
              }
              frame "Brightness  **", "Color Level  **", "Compression  **", "FPS  **", "Sharpness  **" {
                n218 = call <vilib>:"NT Read Number.vi"("Name"=w369) -> ("Numeric"=w368:dbl)  [unwired: 9 in, 1 out]
                n219 = local write "Test Slider"(w368) -> ()
                n220 = property on="Test Slider" class="Slide (strict)"("Visible"=TRUE, "Scale.Maximum"=100.0 ("Scale.Range:Maximum")) -> ()  [unwired: 2 in, 2 out]
                n221 = property on="Test Ring" class="Ring (strict)"("Visible"=FALSE) -> ()  [unwired: 2 in, 2 out]
              }
            }
          }
        }
        n222 = property on="Progress" class="Clust (strict)"("Visible"=FALSE) -> ()  [unwired: 2 in, 2 out]
      }
      event "Test Name": Mouse Enter {
        # "Populate the ring with the list of tests"
        n223 = event-data() -> ()  [unwired: 1 in, 1 out]
        n224 = call <vilib>:"NT Read String Array.vi"("Name"="TestMode/TestList") -> ("String Array"=w377:string[])  [unwired: 9 in, 1 out]
        n225 = Build Array (concatenate)("Select the test to run...", w377) -> (w376:string[])
        n226 = property on="Test Name" class="Ring (strict)"("Strings []"=w376) -> ()  [unwired: 2 in, 2 out]
      }
      event "Test Name": Value Change {
        w379 = FALSE ("Visible")
        # "Tell the robot the test name to run"
        n227 = event-data() -> ("NewVal"=w383:u16)  [unwired: 1 in]
        n228 = property on="Test Name" class="Ring (strict)"() -> ("Strings []"=w384:string[])  [unwired: 2 in, 2 out]
        n229 = local write "Progress"(T6 {"Test Progress"=0, "Test Progress Text"=""} ("Progress")) -> ()
        n230 = Index Array(array=w384, index=w383) -> (element=w382:string)
        n231 = call <vilib>:"NT Write String.vi"("String"=w382, "Name"="TestMode/TestName") -> ()  [unwired: 9 in, 1 out]
        n232 = property on="Progress" class="Clust (strict)"("Visible"=TRUE) -> ()  [unwired: 2 in, 2 out]
        n233 = property on="Motor" class="Clust (strict)"("Visible"=w379) -> ()  [unwired: 2 in, 2 out]
        n234 = property on="Test Slider" class="Slide (strict)"("Visible"=w379) -> ()  [unwired: 2 in, 2 out]
        n235 = property on="On/Off" class="Bool (strict)"("Visible"=w379) -> ()  [unwired: 2 in, 2 out]
        n236 = property on="Rev/Fwd" class="Clust (strict)"("Visible"=w379) -> ()  [unwired: 2 in, 2 out]
        n237 = property on="Test Ring" class="Ring (strict)"("Visible"=w379) -> ()  [unwired: 2 in, 2 out]
      }
      event "Select Auto": Mouse Enter {
        # "Populate the combo box with the list of autonomous options"
        n238 = event-data() -> ()  [unwired: 1 in, 1 out]
        n239 = call <vilib>:"NT Read String Array.vi"("Name"="Auto List") -> ("String Array"=w386:string[])  [unwired: 9 in, 1 out]
        n240 = property on="Select Auto" class="CmbBox"("Strings[]"=w386) -> ()  [unwired: 2 in, 2 out]
      }
      event "Select Auto": Value Change {
        # "User modified the Auto Selection. Write to NT variable so robot knows."
        n241 = event-data() -> ("NewVal"=w389:string)  [unwired: 1 in]
        n242 = call <vilib>:"NT Write String.vi"("String"=w389, "Name"="Auto Selector") -> ()  [unwired: 9 in, 1 out]
      }
      event "Command Selection": Value Change {
        # "Get the params and show in table"
        n243 = event-data() -> ("NewVal"=w395:i32)  [unwired: 1 in]
        n244 = property on="Command Selection" class="MCListbox (strict)"() -> ("ItemNames"=w393:string[][])  [unwired: 2 in, 2 out]
        n245 = call <vilib>:"WPI_DashboardUpdate Command Params.vi"("NewVal"=w395, "Commands"=w393, "Param Tbl"=w394) -> ()  [unwired: 8 in, 1 out]
      }
      event "Execute Command": Value Change {
        # "Started one, Unique ID holds\nresponse"
        n246 = event-data() -> ()  [unwired: 1 in, 1 out]
        n247 = property on="Command Selection" class="MCListbox (strict)"() -> ("ItemNames"=w406:string[][])  [unwired: 2 in, 2 out]
        n248 = Index Array(array=w406, index (row)="Command Selection", index (col)=0) -> (element=w404:string)
        n249 = call <vilib>:"Invoke Commands.vi"("Command Params"="Command Params", "Function Name"=w404) -> ("Params"=w400:u8, "Started"=w399:bool)  [unwired: 7 in, 1 out]
        n250 = Array Subset(array="Command Params", length (row)=w400) -> (w401:string[][])  [unwired: 3 in]
        n251 = Select(t="Executing" ("Cmd Status"), s=w399, f="" ("Cmd Status")) -> (s? t:f=→"Cmd Status":string)
      }
      event "Command Selection": Double Click {
        n252 = event-data() -> ("Row"=w414:i32)  [unwired: 1 in]
        n253 = property on="Command Selection" class="MCListbox (strict)"() -> ("ItemNames"=w417:string[][])  [unwired: 2 in, 2 out]
        n254 = local read "Command Params"() -> (w413:string[][])
        n255 = Index Array(array=w417, index (row)=w414, index (col)=0) -> (element=w415:string)
        n256 = call <vilib>:"Invoke Commands.vi"("Command Params"=w413, "Function Name"=w415) -> ("Params"=w412:u8, "Started"=w407:bool)  [unwired: 7 in, 1 out]
        n257 = Array Subset(array=w413, length (row)=w412) -> (w411:string[][])  [unwired: 3 in]
        n258 = Select(t="Executing" ("Cmd Status"), s=w407, f="" ("Cmd Status")) -> (s? t:f=w408:string)
        n259 = local write "Cmd Status"(w408) -> ()
      }
      event "CheckList": Double Click {
        # "Shift clears all"
        # "Update symbols on the listbox"
        n260 = event-data() -> ("PlatMods.Shift"=w419:bool, "Row"=w421:i32)  [unwired: 1 in]
        n261 = case shown="True" w419 {
          tunnel: w421 -> [w425 _]
          tunnel: 1 -> [w424 _]
          frame False {
            n262 = property on="CheckList" class="LstBox (strict)"() -> ("Item Symbols"=w423:i32[])  [unwired: 2 in, 2 out]
            n263 = Replace Array Subset(array=w423, new element=w424, index=w425) -> (w422:i32[])
            n264 = property on="CheckList" class="LstBox (strict)"("Item Symbols"=w422) -> ()  [unwired: 2 in, 2 out]
          }
          frame True {
            w426 = 0 ("Top Row")
            n265 = property on="CheckList" class="LstBox (strict)"() -> ("Number of Rows"=w428:u32)  [unwired: 2 in, 2 out]
            n266 = Initialize Array(0, w428) -> (w427:i32[])
            n267 = property on="CheckList" class="LstBox (strict)"("Top Row"=w426, "Value"=w426, "Item Symbols"=w427) -> ()  [unwired: 2 in, 2 out]
          }
        }
      }
      event "CheckList": Key Down {
        # "Update symbols on the listbox\nLeft and right keys check and uncheck"
        n268 = event-data() -> ("VKey"=w432:T21)  [unwired: 1 in]
        n269 = case shown="\"Left\", \"Right\"" w432 {
          selector: w432 -> [w437 _]
          tunnel: eventvkey."Left" ("VKey") -> [w435 _]
          frame "Left", "Right" {
            n270 = Equal?(x=w435, y=w437) -> (x = y?=w436:bool)
            n271 = Select(t=0, s=w436, f=1) -> (s? t:f=w438:i32)
            n272 = property on="CheckList" class="LstBox (strict)"() -> ("Item Symbols"=w441:i32[])  [unwired: 2 in, 2 out]
            n273 = Replace Array Subset(array=w441, new element=w438, index="CheckList") -> (w440:i32[])
            n274 = property on="CheckList" class="LstBox (strict)"("Item Symbols"=w440) -> ()  [unwired: 2 in, 2 out]
          }
          frame Default {
          }
        }
      }
      event "Motor.Enable": Value Change {
        # "When the test mode otor enable helper is set, update that\ntree row item's value"
        n275 = event-data() -> ("NewVal"=w447:bool)  [unwired: 1 in]
        n276 = Unbundle("Motor") -> ("Value"=w446:dbl)  [unwired: 1 out]
        n277 = Select(t=w446, s=w447, f=0.0) -> (s? t:f=w444:dbl)
        n278 = call <vilib>:"NT Write Number.vi"("Numeric"=w444, "Name"=w443) -> ()  [unwired: 9 in, 1 out]
      }
      event "Test Slider": Value Change {
        # "When the test mode slider helper is set, update that\ntree row item's value"
        n279 = event-data() -> ("NewVal"=w450:dbl)  [unwired: 1 in]
        n280 = call <vilib>:"NT Write Number.vi"("Numeric"=w450, "Name"=w451) -> ()  [unwired: 9 in, 1 out]
      }
      event "On/Off": Value Change {
        # "When the test mode on/off helper value is set, update that\ntree row item's value"
        n281 = event-data() -> ("NewVal"=w455:bool)  [unwired: 1 in]
        n282 = Boolean To (0,1)(Boolean=w455) -> (0, 1=w454:i16)
        n283 = call <vilib>:"NT Write Number.vi"("Numeric"=w454, "Name"=w453) -> ()  [unwired: 9 in, 1 out]
      }
      event "Rev/Fwd": Value Change {
        # "When the test mode helper value for relays is set, update that\ntree row item's value"
        n284 = event-data() -> ("NewVal.Forward"=w463:bool, "NewVal.Reverse"=w462:bool)  [unwired: 1 in]
        n285 = Boolean To (0,1)(Boolean=w463) -> (0, 1=w459:i16)
        n286 = Boolean To (0,1)(Boolean=w462) -> (0, 1=w461:i16)
        n287 = Negate(x=w461) -> (-x=w460:i16)
        n288 = Add(x=w459, y=w460) -> (x+y=w458:i16)
        n289 = call <vilib>:"NT Write Number.vi"("Numeric"=w458, "Name"=w457) -> ()  [unwired: 9 in, 1 out]
      }
      event "Test Ring": Value Change {
        # "When a test mode helper value is selected from the ring,\nset the tree item's variable to the string value"
        n290 = event-data() -> ("NewVal"=w467:u16)  [unwired: 1 in]
        n291 = property on="Test Ring" class="Ring (strict)"() -> ("Strings []"=w468:string[])  [unwired: 2 in, 2 out]
        n292 = Index Array(array=w468, index=w467) -> (element=w466:string)
        n293 = call <vilib>:"NT Write String.vi"("String"=w466, "Name"=w465) -> ()  [unwired: 9 in, 1 out]
      }
      event "Rec Mode": Value Change {
        # "Update globals for recording mode and path to read log from.\nClear when logging and let NetworkTables set path for vision to\nuse."
        n294 = event-data() -> ("NewVal"=w479:enum32{"Stop", "Record", "Playback"})  [unwired: 1 in]
        n295 = global write "WPI_DashboardLogging Global.vi" "Logging Filename"(path "") -> ()
        n296 = global write "WPI_DashboardLogging Global.vi" "Recording"(w479) -> ()
        n297 = case shown="\"Playback\"" w479 {
          tunnel: w478 -> [_ w481 w490]
          tunnel: [_ _ w489] -> w476
          tunnel: [_ _ w488] -> _
          tunnel: w474 -> [_ _ w486]
          tunnel: cluster{i32, i32} {-250, 170} -> [_ _ w485]
          tunnel: [_ _ T22 {"Image Size"=TRUE, "Image Type"=TRUE, "Pixel Value"=TRUE, "ROI Information"=TRUE, "Zoom Factor"=FALSE} ("Image Information Shown:All Elements")] -> w469
          tunnel: [_ _ TRUE ("Zoom Factor")] -> w470
          tunnel: w472 -> [_ _ w482]
          frame Default {
          }
          frame "Stop", "Record" {
            # "Place Window too"
            n298 = invoke class="VI" method="FP.Close"(reference=w481) -> (reference out=w480:refnum<vi>)  [unwired: 2 in, 2 out]
            n299 = invoke class="VI" method="Abort VI"(reference=w480) -> ()  [unwired: 2 in, 3 out]
          }
          frame "Playback" {
            n300 = call "Open Playback Panel.vi"("Offset"=w485, "DB VI Ref"=w486, "Playback in"=w490) -> ("Playback out"=w487:refnum<vi>)  [unwired: 8 in]
            n301 = register-events(w487, w482) -> (reference out=w489:refnum<event-registration>, error out=w488:errorcluster)  [unwired: 2 in]
          }
        }
        n302 = property on="Camera Image Right" class="ImageControl"("Image Information Shown"=w469, "Image Information Visible"=w470) -> ()  [unwired: 2 in, 2 out]
        n303 = property on="Camera Image" class="ImageControl"("Image Information Shown"=w469, "Image Information Visible"=w470) -> ()  [unwired: 2 in, 2 out]
        n304 = call <vilib>:"WPI_DashboardNT Log FieldName Cache.vi"("Operation"=enum16{"Lookup/Add", "Index", "Clear"}."Clear") -> ()  [unwired: 8 in, 3 out]
      }
      event Panel Close {
        w492 = enum32{"Stop", "Record", "Playback"}."Stop" ("Rec Mode")
        # "Playback window has been closed, abort"
        n305 = event-data() -> ()  [unwired: 1 in, 4 out]
        n306 = local write "Rec Mode"(w492) -> ()
        n307 = global write "WPI_DashboardLogging Global.vi" "Recording"(w492) -> ()
      }
      event Panel Close {
        # "Abort playback window and ourself"
        n308 = event-data() -> ()  [unwired: 1 in, 4 out]
        n309 = invoke class="VI" method="FP.Close"(reference=w496) -> (reference out=w495:refnum<vi>)  [unwired: 2 in, 2 out]
        n310 = invoke class="VI" method="Abort VI"(reference=w495) -> (error out=w494:errorcluster)  [unwired: 2 in, 2 out]
        n311 = invoke class="VI" method="Abort VI"(error in=w494) -> ()  [unwired: 2 in, 3 out]
      }
      event User Event {
        n312 = event-data() -> ("IDs"=w503:cluster{"RPC field ID":u16, "Unique ID":u16}, "String"=w502:string)  [unwired: 1 in]
        n313 = Bundle("IDs"=w503, "String"=w502) -> (w501:T9)  [unwired: 1 in]
        n314 = call <vilib>:"Retrieve RPC Response.vi"("RPC Response"=w501) -> ("Output"=w499:string[][])  [unwired: 10 in]
        n315 = Build Array (concatenate)(w497, w499) -> (w498:string[][])
        n316 = local write "Command Params"(w498) -> ()
        n317 = local write "Cmd Status"("" ("Cmd Status")) -> ()
      }
      event "Tree": Double Click {
        n318 = event-data() -> ("PlatMods"=w509:T25, "Tag"=w506:string)  [unwired: 1 in]
        n319 = Unbundle(w509) -> ("Shift"=w508:bool)  [unwired: 4 out]
        n320 = String Subset(string=w506, length (rest)=1 ("length (rest)")) -> (substring=w505:string)  [unwired: 1 in]
        n321 = Not(x=w508) -> (.not. x?=w507:bool)
        n322 = case shown="\"/\"" w505 {
          tunnel: w506 -> [_ w512]
          tunnel: w507 -> [_ w511]
          frame Default {
          }
          frame "/" {
            n323 = call <vilib>:"NT Update Persistence.vi"("Persistence"=w511, "Name"=w512) -> ()  [unwired: 9 in, 1 out]
          }
        }
      }
    }
  }
  n324 = while {
    tunnel: w65 -> [w514]
    i -> [w517]
    stop <- FALSE stop-if-true
    n325 = Wait (ms)(milliseconds to wait=u32 100) -> ()  [unwired: 1 out]
    n326 = case shown="\"Playback\"" "Rec Mode" {
      tunnel: w517 -> [_ _ w532]
      tunnel: [u32 2829099 ("Base Color") u32 11141120 ("Target Color") w521] -> w513
      frame "Stop", Default {
        # "Reset the color, extra updates don't cost much"
      }
      frame "Record" {
      }
      frame "Playback" {
        # "Playback"
        n327 = Quotient & Remainder(x=w532, y=u32 50 ("milliseconds to wait")) -> (x-y*floor(x/y)=w528:u32)  [unwired: 1 out]
        n328 = Divide(x=w528, y=u32 50 ("milliseconds to wait")) -> (x/y=w525:dbl)
        n329 = Multiply(x=6.283185307179586, y=w525) -> (x*y=w530:dbl)
        n330 = Sine(x=w530) -> (sin(x)=w529:dbl)
        n331 = Absolute Value(x=w529) -> (abs(x)=w522:dbl)
        n332 = call "Interpolate RGB Color.vi"("Proportion"=w522, "Target Color"=u32 30976, "Base Color"=u32 2829099) -> ("Result Color"=w521:u32)  [unwired: 8 in]
      }
    }
    n333 = property class="Pane"(reference=w514, "PaneColor"=w513) -> ()  [unwired: 1 in, 2 out]
  }
  n334 = local write "Dashboard Tab"(T2."Drive" ("Dashboard Tab")) -> ()
  n335 = property on="On/Off" class="Bool (strict)"("Visible"=w36) -> ()  [unwired: 2 in, 2 out]
  n336 = property on="Motor" class="Clust (strict)"("Visible"=w36) -> ()  [unwired: 2 in, 2 out]
  n337 = property on="Progress" class="Clust (strict)"("Visible"=w36) -> ()  [unwired: 2 in, 2 out]
  n338 = property on="Test Ring" class="Ring (strict)"("Visible"=w36) -> ()  [unwired: 2 in, 2 out]
  n339 = property on="Rev/Fwd" class="Clust (strict)"("Visible"=w36) -> ()  [unwired: 2 in, 2 out]
  n340 = while {
    tunnel: u16 1741 ("timeout ms (25000)") -> [w534]
    stop <- FALSE stop-if-true
    n341 = TCP Create Listener(10:w534) -> (0:w533:errorcluster, 3:w535:refnum<k5>)  [unwired: 4 in, 1 out]
    n342 = case shown="No Error" w533 {
      selector: w533 -> [w537 _]
      tunnel: w535 -> [w538 _]
      frame No Error {
        n343 = while {
          tunnel: w538 -> [w541]
          tunnel: w537 -> [w540]
          stop <- FALSE stop-if-true
          n344 = TCP Wait On Listener(8:w540, 11:w541) -> (0:w542:errorcluster, 4:w543:refnum<k5>)  [unwired: 2 in, 3 out]
          n345 = local write "TCP"(w543) -> ()
          n346 = case shown="No Error" w542 {
            frame No Error {
            }
            frame Error {
              n347 = Wait (ms)(milliseconds to wait=u32 1000) -> ()  [unwired: 1 out]
            }
          }
        }
      }
      frame Error {
        n348 = Wait (ms)(milliseconds to wait=u32 1000) -> ()  [unwired: 1 out]
      }
    }
  }
  n349 = local write "Command Selection"(u16 0 ("milliseconds to wait")) -> ()
  n350 = local write "Command Params"(string[][] [] ("Command Params")) -> ()
  n351 = global write "WPI_DashboardLogging Global.vi" "Recording"(w59) -> ()
  n352 = local write "Rec Mode"(w59) -> ()
  n353 = call <vilib>:"NT Write String.vi"("String"="Select Auto", "Name"="Auto Selector") -> ()  [unwired: 9 in, 1 out]
